vi "Cmd Get Binary Parameter Value (C).vi"(6 "error in (no error)":errorcluster, 7 "type":variant, 8 "parameter index":variant, 9 "command reference":T1) -> (0 "error out":errorcluster, 1 "value":variant, 3 "command reference out":T1)   [LabVIEW 2012, in "NI_Database_API_64.lvlib"]
doc: "Retrieves the value of the parameter specified by the <B>parameter index</B> input in the command or command-recordset. The <B>parameter index</B> can be either the zero-indexed position of the parameter in the command or the name of the parameter. Wire data to the <B>type</B> input to determine the polymorphic instance to use or manually select the instance."
uses:
  NI_Database_API_64.lvlib
  Cmd ObjectReference.ctl
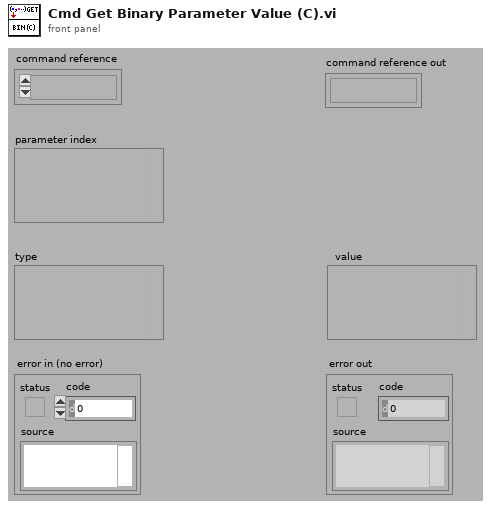
[diagram p1: front panel]
types:
  T1 = typedef "NI_Database_API_64.lvlib/Cmd ObjectReference.ctl" = refnum<k1>
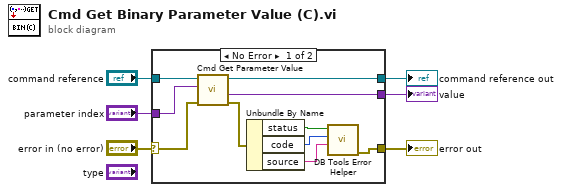
[diagram p0: block diagram]
diagram:
  n1 = case shown="No Error" "error in (no error)" {
    selector: "error in (no error)" -> [w7 w18]
    tunnel: "parameter index" -> [w16 _]
    tunnel: [w15 _] -> w5
    tunnel: "command reference" -> [w14 w17]
    tunnel: [w13 w17] -> w3
    tunnel: [w8 w18] -> w2
    frame No Error {
      n2 = call "Cmd Get Parameter Value.vi"("error in (no error)"=w7, "parameter index"=w16, "command reference"=w14) -> ("error out"=w9:errorcluster, "value"=w15:variant, "command reference out"=w13:T1)  [unwired: 2 out]
      n3 = Unbundle By Name(w9) -> ("status"=w11:bool, "code"=w10:i32, "source"=w12:string)
      n4 = call "DB Tools Error Helper.vi"("source"=w12, "code"=w10, "status"=w11) -> ("error out"=w8:errorcluster)  [unwired: 1 in, 7 out]
    }
    frame Error {
    }
  }
  "error out" <- w2
  "command reference out" <- w3
  "value" <- w5
